vi "IEEE754 Integer to SGL.vi"(7 "ieee 754 integer":fxp<+,32,32>=1031798784.0 format="%.0b") -> (8 "SGL":sgl=92.92 format="%.10f")   [LabVIEW 2010]
panel:
  out "Mantissa":dbl=1.4518749713897705 format="%.8f"
  out "Exponent":i32=6
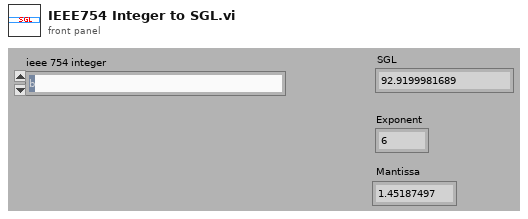
[diagram p1: front panel]
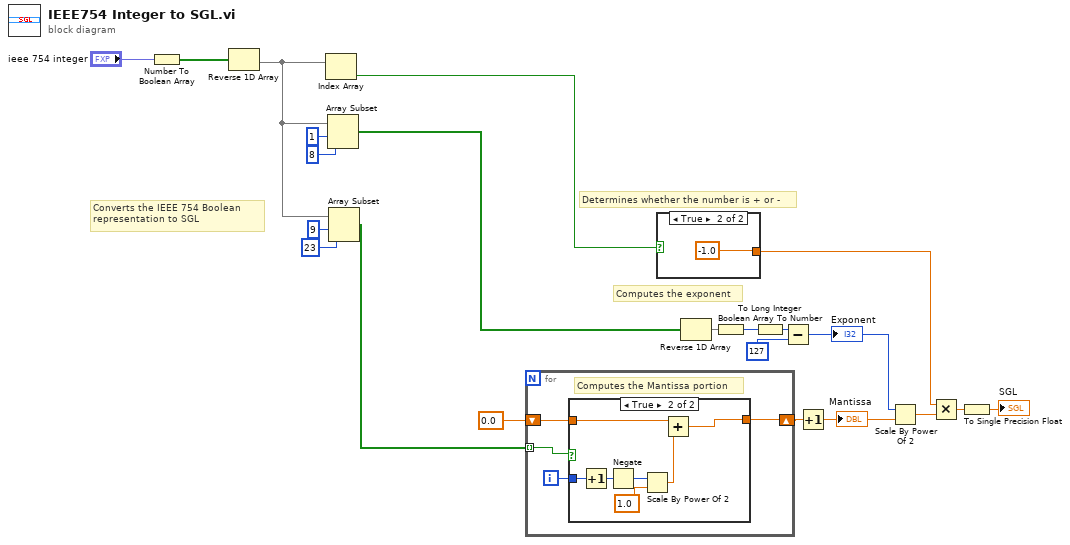
[diagram p0: block diagram]
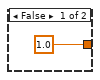
[diagram p2: hidden frame]
diagram:
  # "Computes the exponent"
  # "Determines whether the number is + or -"
  # "Converts the IEEE 754 Boolean \nrepresentation to SGL"
  n1 = Number To Boolean Array(number="ieee 754 integer") -> (Boolean array=w21:bool[])
  n2 = Reverse 1D Array(array=w21) -> (reversed array=w2:bool[])
  n3 = Index Array(array=w2) -> (element=w6:bool)  [unwired: 1 in]
  n4 = Array Subset(array=w2, index=1, length=8) -> (w5:bool[])
  n5 = Array Subset(array=w2, index=9, length=23) -> (w1:bool[])
  n6 = for {
    tunnel: w1 -> [w26] mode=indexing
    shift-right: [w23] -> w8
    shift-left: 0.0 -> [w24]
    i -> [w25]
    # "Computes the Mantissa portion"
    n7 = case shown="True" w26 {
      tunnel: w25 -> [_ w34]
      tunnel: w24 -> [w27 w30]
      tunnel: [w27 w28] -> w23
      frame False {
      }
      frame True {
        n8 = Increment(x=w34) -> (x+1=w33:i32)
        n9 = Negate(x=w33) -> (-x=w32:i32)
        n10 = Scale By Power Of 2(n=w32, x=1.0) -> (x*2^n=w29:dbl)
        n11 = Add(x=w30, y=w29) -> (x+y=w28:dbl)
      }
    }
  }
  n12 = case shown="True" w6 {
    tunnel: [1.0 -1.0] -> w14
    frame False {
    }
    frame True {
    }
  }
  n13 = Reverse 1D Array(array=w5) -> (reversed array=w12:bool[])
  n14 = Boolean Array To Number(Boolean array=w12) -> (number=w16:u32)
  n15 = To Long Integer(number=w16) -> (32bit integer=w17:i32)
  n16 = Subtract(x=w17, y=127) -> (x-y=w15:i32)
  "Exponent" <- w15
  n17 = Increment(x=w8) -> (x+1=w10:dbl)
  "Mantissa" <- w10
  n18 = Scale By Power Of 2(n=w15, x=w10) -> (x*2^n=w11:dbl)
  n19 = Multiply(x=w14, y=w11) -> (x*y=w13:dbl)
  n20 = To Single Precision Float(number=w13) -> (single precision float=→"SGL":sgl)
